vi "leftarm11109.vi"() -> ()   [LabVIEW 2017]
uses:
  <vilib>/MakerHub/LINX/Public/Utilities/Open Serial.vi
  <vilib>/MakerHub/LINX/Public/Sensors/Motion/Servo/Servo Open N Channels.vi
  global variable.vi
  <vilib>/MakerHub/LINX/Public/Sensors/Motion/Servo/Servo Set Pulse Width N Channels.vi
  <vilib>/MakerHub/LINX/Public/Sensors/Motion/Servo/Servo Close N Channels.vi
  <vilib>/MakerHub/LINX/LMH-LINX.lvlib
  <vilib>/MakerHub/LINX/Public/Sensors/Motion/Servo/Servo.lvlib
panel:
  out "Pulse Widths (uS) 2":u16[](array[numeric])
  in  "Servo Channels":u8[](array[numeric])
  in  "Serial Port":refnum<visa-resource-name>="N/A"
  in  "Stop Button":bool
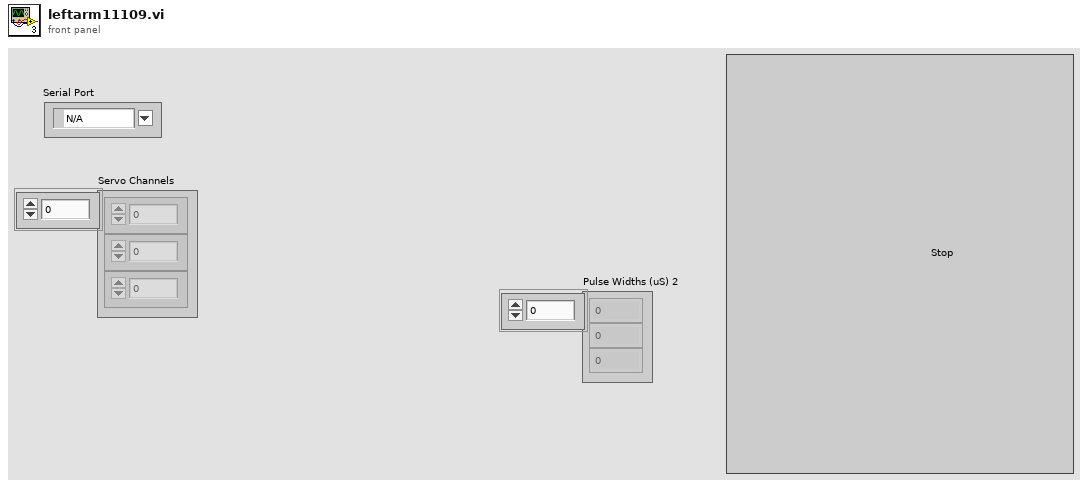
[diagram p1: front panel]
types:
  T1 = typedef "LMH-LINX.lvlib/LINX Ref.ctl" = cluster{"IO":T2, "Interface":T3, "LINX Device Config":T4}
  T2 = typedef "LMH-LINX.lvlib/Platform.ctl" = enum16{"Remote", "Local"}
  T3 = typedef "LMH-LINX.lvlib/Interface.ctl" = enum16{"Serial", "TCP"}
  T4 = typedef "LMH-LINX.lvlib/Device.lvlib/LINX Device Config.ctl" = cluster{"Interface":T3, "COM Port":refnum<visa-resource-name>, "TCP Configuration":T5, "Device Family":u8, "Device ID":u8, "Device Name":string, "TCP Ref":refnum<k5>, "Channels":T6}
  T5 = typedef "LMH-LINX.lvlib/Device.lvlib/TCP Config.ctl" = cluster{"IP Address":string, "Port":u16}
  T6 = typedef "LMH-LINX.lvlib/Channels.ctl" = cluster{"DI":u8[], "DO":u8[], "AI":u8[], "AO":u8[], "PWM":u8[], "QE":u8[], "UART":u8[], "I2C 2":u8[], "SPI":u8[], "CAN":u8[], "Servo":u8[], "AI Ref (V)":dbl, "AI Resolution (Bits)":u8, "AO Ref (V)":dbl, "AO Resolution (Bits)":u8}
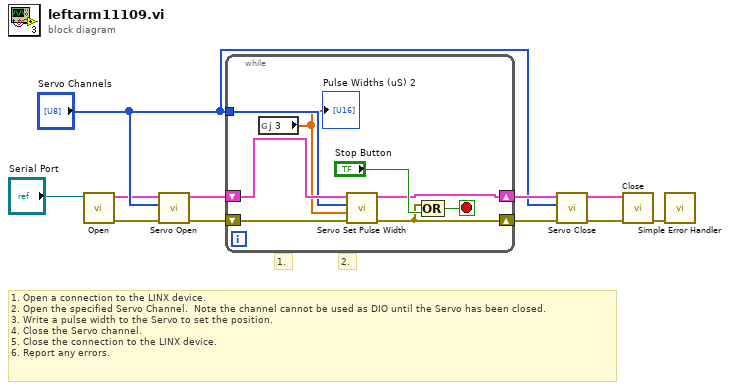
[diagram p0: block diagram]
diagram:
  # "1. Open a connection to the LINX device.\n2. Open the specified Servo Channel.  Note the channel cannot be used as DIO until the Servo has been closed.\n3. Write a pulse width to the Servo to set the position.\n4. Close the Servo channel.  \n5. Close the connection to the LINX device.\n6. Report any errors."
  # "2."
  # "1."
  n1 = call-poly <vilib>:"Open.vi"("Serial Port"="Serial Port") -> ("Error Out"=w11:errorcluster, "LINX Resource"=w1:T1)  [unwired: 8 in, 1 out]
  n2 = call-poly <vilib>:"Servo Open.vi"("Error In"=w11, "Servo Channels"="Servo Channels", "LINX Resource"=w1) -> ("Error Out"=w10:errorcluster, "LINX Resource"=w9:T1)  [unwired: 7 in]
  n3 = while {
    shift-right: [w16] -> w4
    shift-left: w10 -> [w17]
    shift-right: [w14] -> w7
    shift-left: w9 -> [w15]
    tunnel: "Servo Channels" -> [w13]
    stop <- w19 stop-if-true
    n4 = global read "global variable.vi" "j 3"() -> (w12:dbl[])
    "Pulse Widths (uS) 2" <- w12
    n5 = call-poly <vilib>:"Servo Set Pulse Width.vi"("Error In"=w17, "Pulse Widths (uS)"=w12, "Servo Channels"=w13, "LINX Resource"=w15) -> ("Error Out"=w16:errorcluster, "LINX Resource"=w14:T1)  [unwired: 6 in]
    n6 = Compound Arithmetic op=OR ("복합 연산")(w16, "Stop Button") -> (w19:bool)
  }
  n7 = call-poly <vilib>:"Servo Close.vi"("Error In"=w4, "Servo Channels"="Servo Channels", "LINX Resource"=w7) -> ("Error Out"=w5:errorcluster, "LINX Resource"=w6:T1)  [unwired: 7 in]
  n8 = call <vilib>:"Close.vi"("Error In"=w5, "LINX Resource"=w6) -> ("Error Out"=w8:errorcluster)  [unwired: 9 in]
  n9 = call <vilib>:"Simple Error Handler.vi"("error in (no error)"=w8) -> ()  [unwired: 4 in, 5 out]
